vi "DAQ Test_DLL.vi"(7 "rate":dbl=1000.0, 8 "error in":errorcluster, 9 "Time":dbl, 10 "data":dynamicdata(waveform), 11 "device name":tag="cDAQ2Mod1") -> (0 "error out":errorcluster, 3 "task out":refnum<k21>)   [LabVIEW 2015]
uses:
  <vilib>/DAQmx/write.llb/DAQmx Write (Analog 1D Wfm NChan NSamp).vi
  <vilib>/DAQmx/create/channels.llb/DAQmx Create Channel (AO-Voltage-Basic).vi
  <vilib>/DAQmx/configure/timing.llb/DAQmx Timing (Sample Clock).vi
  <vilib>/DAQmx/miscellaneous.llb/DAQmx Fill In Error Info.vi
  <resource>/objmgr/daqmx.rc
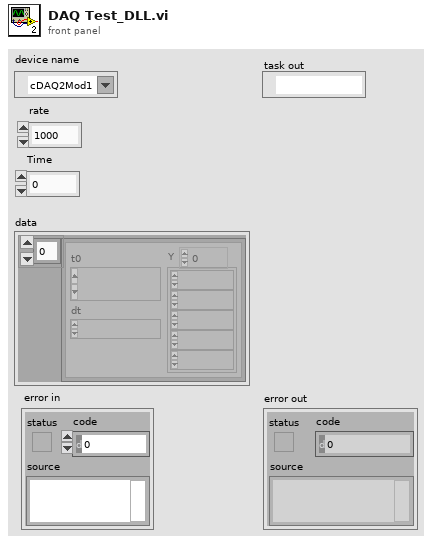
[diagram p1: front panel]
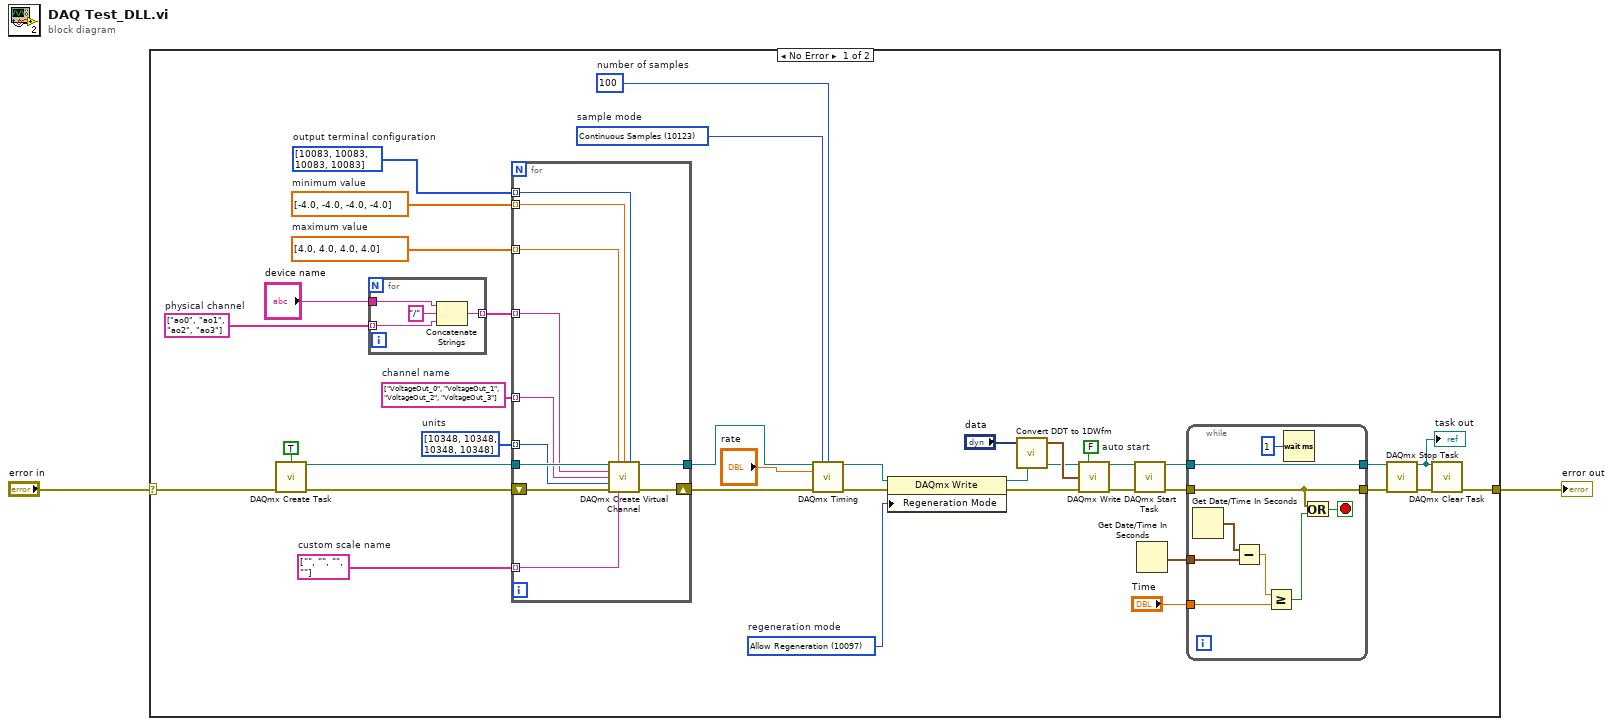
[diagram p0: block diagram]
diagram:
  n1 = case shown="No Error" "error in" {
    selector: "error in" -> [w5 w64]
    tunnel: [w6 w64] -> w2
    frame No Error {
      w16 = FALSE  # auto start
      w21 = 10097 items=["Allow Regeneration"=10097, "Do Not Allow Regeneration"=10158]  # regeneration mode
      w24 = 10123 items=["Finite Samples"=10178, "Continuous Samples"=10123, "Hardware Timed Single Point"=12522]  # sample mode
      w26 = 100  # number of samples
      w29 = i32[] [10083, 10083, 10083, 10083] items=["Default"=-1, "RSE"=10083, "Differential"=10106, "Pseudodifferential"=12529]  # output terminal configuration
      w30 = string[] ["", "", "", ""]  # custom scale name
      w31 = i32[] [10348, 10348, 10348, 10348] items=["Volts"=10348, "From Custom Scale"=10065]  # units
      w32 = string[] ["VoltageOut_0", "VoltageOut_1", "VoltageOut_2", "VoltageOut_3"]  # channel name
      w34 = dbl[] [4.0, 4.0, 4.0, 4.0]  # maximum value
      w35 = dbl[] [-4.0, -4.0, -4.0, -4.0]  # minimum value
      w38 = string[] ["ao0", "ao1", "ao2", "ao3"]  # physical channel
      n2 = call <vilib>:"DAQmx Create Task.vi"("auto cleanup"=TRUE, "error in"=w5) -> ("task out"=w37:refnum<k21>, "error out"=w36:errorcluster)  [unwired: 12 in]
      n3 = for {
        tunnel: [w43] -> w33 mode=indexing
        tunnel: "device name" -> [w42]
        tunnel: w38 -> [w40] mode=indexing
        n4 = Concatenate Strings(w42, "/" ("string"), w40) -> (w43:string)
      }
      n5 = for {
        tunnel: w37 -> [w63]
        tunnel: [w61] -> w28
        tunnel: w35 -> [w59] mode=indexing
        tunnel: w34 -> [w58] mode=indexing
        tunnel: w33 -> [w57] mode=indexing
        tunnel: w32 -> [w56] mode=indexing
        tunnel: w31 -> [w55] mode=indexing
        tunnel: w30 -> [w54] mode=indexing
        shift-right: [w60] -> w27
        shift-left: w36 -> [w62]
        tunnel: w29 -> [w53] mode=indexing
        n6 = call-poly <vilib>:"DAQmx Create Virtual Channel.vi"("task in"=w63, "maximum value"=w58, "minimum value"=w59, "output terminal configuration"=w53, "physical channels"=w57, "name to assign"=w56, "units"=w55, "error in"=w62, "custom scale name"=w54) -> ("task out"=w61:refnum<k21>, "error out"=w60:errorcluster)  [unwired: 5 in]
      }
      n7 = call-poly <vilib>:"DAQmx Timing.vi"("task/channels in"=w28, "sample mode"=w24, "samples per channel"=w26, "rate"="rate", "error in"=w27) -> ("task out"=w23:refnum<k21>, "error out"=w22:errorcluster)  [unwired: 9 in]
      n8 = property class="DAQmx Write"(reference=w23, error in=w22, "Regeneration Mode"=w21) -> (reference out=w12:refnum<k21>, error out=w13:errorcluster)
      n9 = call <vilib>:"Convert DDT to 1DWfm.vi"("Dynamic Data Type"="data") -> ("Array of Waveforms"=w18:waveform(dbl)[])  [unwired: 3 in]
      n10 = call-poly <vilib>:"DAQmx Write.vi"("task/channels in"=w12, "auto start"=w16, "data"=w18, "error in"=w13) -> ("task out"=w14:refnum<k21>, "error out"=w15:errorcluster)  [unwired: 9 in, 1 out]
      n11 = call <vilib>:"DAQmx Start Task.vi"("task/channels in"=w14, "error in"=w15) -> ("task out"=w11:refnum<k21>, "error out"=w9:errorcluster)  [unwired: 12 in]
      n12 = Get Date/Time In Seconds() -> (seconds since 1Jan1904=w4:timestamp)
      n13 = while {
        tunnel: w11 -> [w52]
        tunnel: [w52] -> w10
        tunnel: w9 -> [w50]
        tunnel: [w50] -> w8
        tunnel: w4 -> [w47]
        tunnel: "Time" -> [w45]
        stop <- w51 stop-if-true
        n14 = Get Date/Time In Seconds() -> (seconds since 1Jan1904=w48:timestamp)
        n15 = Subtract(x=w48, y=w47) -> (x-y=w46:dbl)
        n16 = Greater Or Equal?(x=w46, y=w45) -> (x >= y?=w44:bool)
        n17 = Wait (ms)(milliseconds to wait=u32 1) -> ()  [unwired: 1 out]
        n18 = Or(x=w50, y=w44) -> (x .or. y?=w51:bool)
      }
      n19 = call <vilib>:"DAQmx Stop Task.vi"("task/channels in"=w10, "error in"=w8) -> ("task out"=w7:refnum<k21>, "error out"=w20:errorcluster)  [unwired: 12 in]
      "task out" <- w7
      n20 = call <vilib>:"DAQmx Clear Task.vi"("task in"=w7, "error in"=w20) -> ("error out"=w6:errorcluster)  [unwired: 13 in]
    }
    frame Error {
    }
  }
  "error out" <- w2
